vi "LWXPS_WaitMotionEnd.vi"(0 "XPS Reference IN":refnum<k24>, 5 "Time out in milliseconds":dbl, 7 "Y position in microns":dbl, 9 "X position in microns":dbl, 11 "LabVIEW error IN":errorcluster) -> (4 "XPS Reference OUT":refnum<k24>, 6 "Returned error code":i32, 8 "XPS Error String":string, 15 "LabVIEW error OUT":errorcluster)   [LabVIEW 2014]
uses:
  D:/XPSQ8_LabView_Library/Development/Source/Dll/Newport.XPS.CommandInterface.dll
  Dll/Newport.XPS.CommandInterface.dll
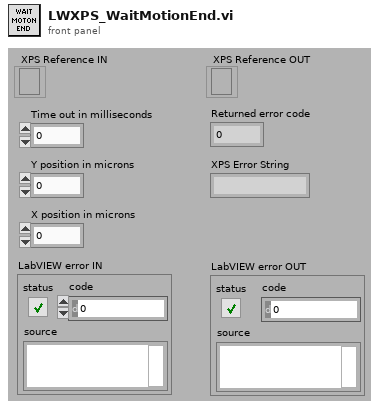
[diagram p1: front panel]
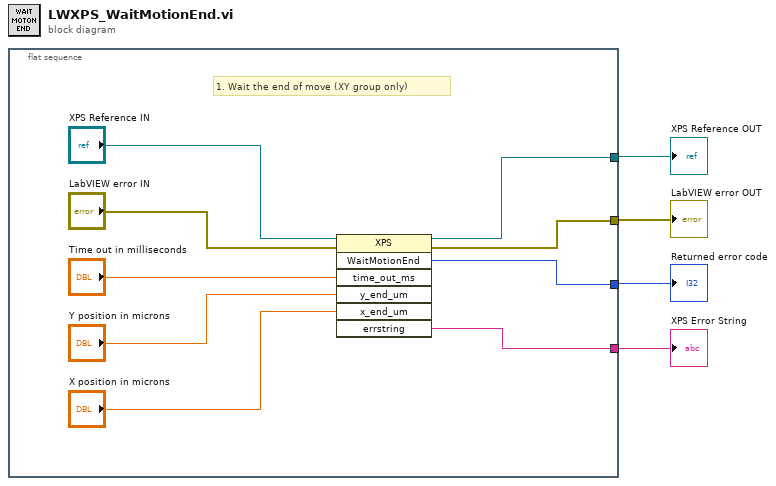
[diagram p0: block diagram]
diagram:
  n1 = flat-sequence {
    tunnel: [w10] -> w4
    tunnel: [w9] -> w3
    tunnel: [w11] -> w2
    tunnel: [w8] -> w1
    frame #0 {
      # "1. Wait the end of move (XY group only)"
      n2 = invoke class="XPS" method="WaitMotionEnd"(reference="XPS Reference IN", error in="LabVIEW error IN", "time_out_ms"="Time out in milliseconds", "y_end_um"="Y position in microns", "x_end_um"="X position in microns") -> (reference out=w10:refnum<k24>, error out=w9:errorcluster, "WaitMotionEnd"=w11:i32, "errstring"=w8:string)  [unwired: 2 in, 3 out]
    }
  }
  "XPS Error String" <- w1
  "XPS Reference OUT" <- w4
  "LabVIEW error OUT" <- w3
  "Returned error code" <- w2
